vi "Kinesis - KPZ101 KSG101 - Set Position.vi"() -> ()   [LabVIEW 2012]
uses:
  U:/Kinesis LabVIEW Website Examples/Thorlabs.MotionControl.Controls.dll
  Thorlabs.MotionControl.Controls.dll
  U:/Kinesis LabVIEW Website Examples/Thorlabs.MotionControl.KCube.PiezoCLI.dll
  Thorlabs.MotionControl.KCube.PiezoCLI.dll
  U:/Kinesis LabVIEW Website Examples/Thorlabs.MotionControl.GenericPiezoCLI.dll
  Thorlabs.MotionControl.GenericPiezoCLI.dll
  U:/Kinesis LabVIEW Website Examples/ThorLabs.MotionControl.KCube.StrainGaugeCLI.dll
  ThorLabs.MotionControl.KCube.StrainGaugeCLI.dll
panel:
  in  "HubMode":i32(ring)=1 items=["AnalogueCh1"=1, "AnalogueCh2"=2, "ExtSignalSMA"=3]
  in  "stop":bool
  in  "Open Loop\nVoltage":dbl
  in  "Close Loop\n% Travel":dbl
  in  "?":bool
  in  "Zero":bool
  in  "Select Mode":bool
  in  "mode":i32(ring)=1 items=["OpenLoop"=1, "CloseLoop"=2, "OpenLoopSmooth"=3, "CloseLoopSmooth"=4]
  in  "KSG101 SerialNumber":string
  in  "KCubeStrainGaugeControl":refnum<k24>(container)
  in  "KPZ101 SerialNumber":string
  in  "KCubePiezoControl":refnum<k24>(container)
  # "Thorlabs Hardware: \nKPZ101 - K-Cube Piezo Controller\nhttps://www.thorlabs.com/newgrouppage9.cfm?objectgroup_id=2421\n\nKSG101 - K-Cube Strain Gauge Controller\nhttps://www.thorlabs.com/newgrouppage9.cfm?objectgroup_ID=242\n\nDescription: This VI will connect to & manage Closed Loop operation of the KPZ101 when used with the KSG101 Strain Gauge Controller.\nIn Closed Loop operation, as piezo actuators show a certain amount of nonlinearity, hysteresis, temperature dependence and aging, a position sensor, in this case a Strain Gauge, is read by KSG101 & feedback position information through a PI loop is managed by KPZ101 to account for this behaviour.  \nWhen in Open Loop mode, the user can adjust the Voltage of the piezo stack. \nWhen in Closed Loop mode, position can be set by use of the SetPercentageTravel() function.\n\nTo explore how to configure the KPZ101 for Closed Loop operation, plaese visit the KPZ101 User Manual. \n https://www.thorlabs.com/thorproduct.cfm?partnumber=KPZ101\n\nInstructions:\n1) Connect your KPZ101 & KSG101 devices to your PC & power each device ensuring these are correctly interconnected. Depending on whether these are connected through the KCH*** K-Cube Hub or via SMA cable will impact the choice of settings below. \nFor full device setup, the device product manual can be found on our website here. - https://www.thorlabs.com/thorproduct.cfm?partnumber=KPZ101\n2) Enter the device serial numbers below.\n3) Click 'Run' in the LabVIEW Toolbar.\n4) Ensure the HubMode is set correctly depending on how your KPZ101 & KSG101 are connected.\n5) Zero each device using the ZERO button.\n6) To end the program, click END PROGRAM."
  # "Notes:"
  # "- Ensure that the appropriate .DLLs are copied into your Project Folder. Check that the correct bit type are used depending on your version of LabVIEW\ni.e. 32-bit or 64-bit.\n\n\n\n\n\n\n\n\n\n\n\n\n\n\n- Open the example VI through the LabVIEW Project Explorer to correctly load the User Interface from Thorlabs.MotionControl.Controls.dll."
  # "Example Image of .NET Controller - VI opened via Project Explorer/ not opened via Project Explorer"
  # "VI Not Opened via Project Explorer"
  # "VI Opened via Project Explorer"
  # "- To explore the range of methods available, please visit the .NET API, included with your Kinesis software.\n\n- For tips on building your own VIs with Thorlabs Motion Control Hardware, please see our LabVIEW Guide here.\nhttps://www.thorlabs.com/newgrouppage9.cfm?objectgroup_id=10285"
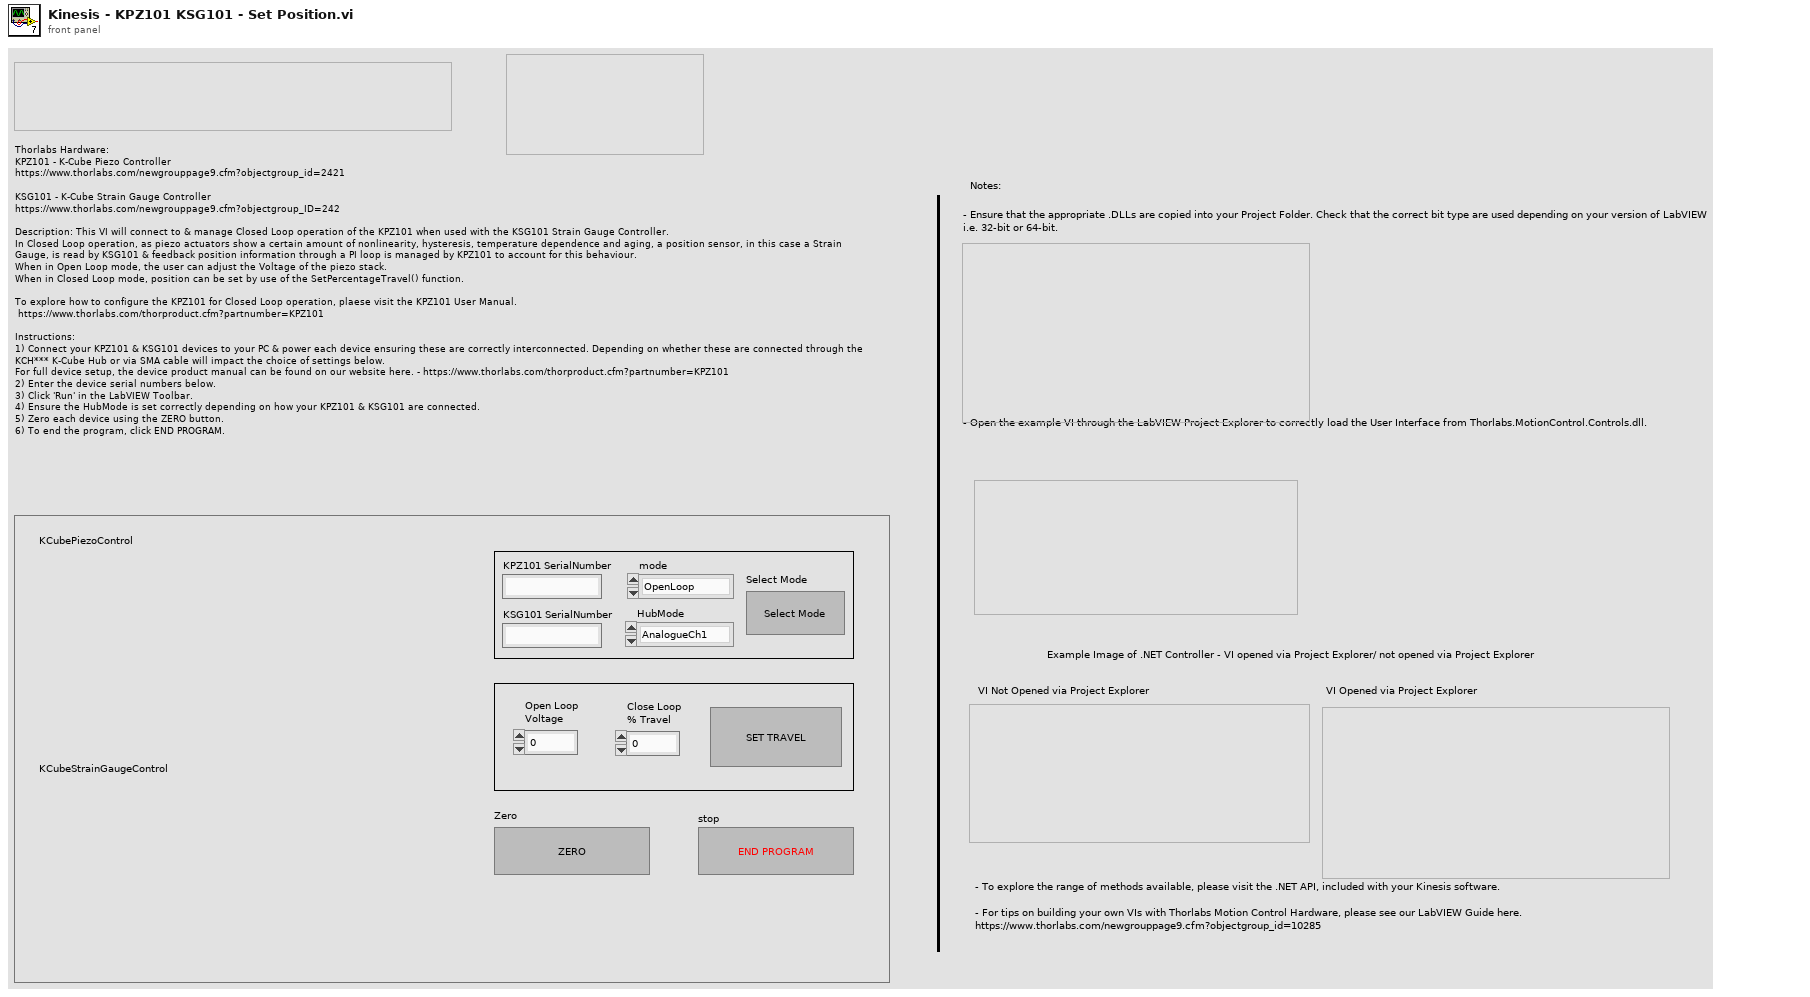
[diagram p1: front panel]
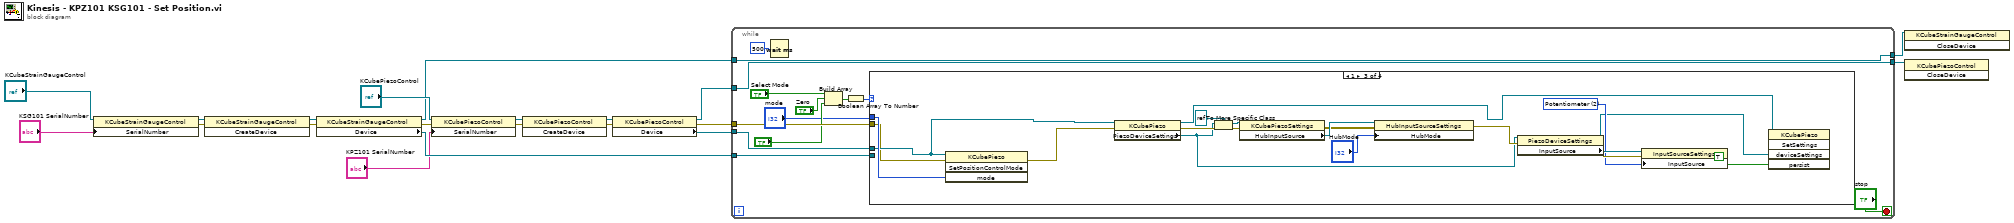
[diagram p0: block diagram]
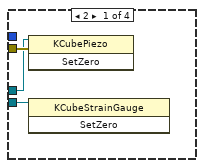
[diagram p2: hidden frame]
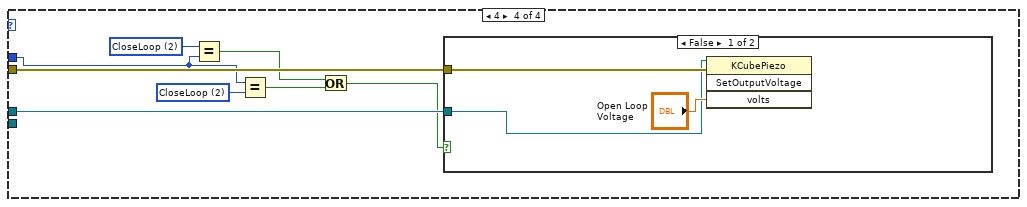
[diagram p4: hidden frame]
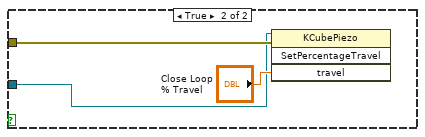
[diagram p5: hidden frame]
diagram:
  n1 = property class="KCubeStrainGaugeControl"(reference="KCubeStrainGaugeControl", "SerialNumber"="KSG101 SerialNumber") -> (reference out=w14:refnum<k24>, error out=w13:errorcluster)  [unwired: 1 in]
  n2 = invoke class="KCubeStrainGaugeControl" method="CreateDevice"(reference=w14, error in=w13) -> (reference out=w12:refnum<k24>, error out=w11:errorcluster)  [unwired: 1 in, 1 out]
  n3 = property class="KCubeStrainGaugeControl"(reference=w12, error in=w11) -> (reference out=w1:refnum<k24>, error out=w9:errorcluster, "Device"=w10:refnum<k24>)
  n4 = property class="KCubePiezoControl"(reference="KCubePiezoControl", error in=w9, "SerialNumber"="KPZ101 SerialNumber") -> (reference out=w17:refnum<k24>, error out=w8:errorcluster)
  n5 = invoke class="KCubePiezoControl" method="CreateDevice"(reference=w17, error in=w8) -> (reference out=w20:refnum<k24>, error out=w19:errorcluster)  [unwired: 1 in, 1 out]
  n6 = property class="KCubePiezoControl"(reference=w20, error in=w19) -> (reference out=w3:refnum<k24>, error out=w7:errorcluster, "Device"=w5:refnum<k24>)
  n7 = while {
    tunnel: w10 -> [w33]
    tunnel: w7 -> [w30]
    tunnel: w5 -> [w24]
    tunnel: [w23] -> w4
    tunnel: w3 -> [w23]
    tunnel: [w22] -> w2
    tunnel: w1 -> [w22]
    stop <- "stop" stop-if-true
    n8 = Wait (ms)(milliseconds to wait=u32 500) -> ()  [unwired: 1 out]
    n9 = Build Array("Select Mode", "Zero", "?") -> (w28:bool[])
    n10 = Boolean Array To Number(Boolean array=w28) -> (number=w26:u32)
    n11 = case shown="1" w26 {
      tunnel: w33 -> [w36 _ _ _]
      tunnel: "mode" -> [_ _ w42 w60]
      tunnel: w30 -> [w35 _ w38 w63]
      tunnel: w24 -> [w34 _ w39 w62]
      frame 2 {
        n12 = invoke class="KCubePiezo" method="SetZero"(reference=w34, error in=w35) -> ()  [unwired: 1 in, 3 out]
        n13 = invoke class="KCubeStrainGauge" method="SetZero"(reference=w36) -> ()  [unwired: 2 in, 3 out]
      }
      frame 0, Default {
      }
      frame 1 {
        w46 = 2 items=["SoftwareOnly", "ExternalSignal", "Potentiometer"] ("InputSource")
        n14 = invoke class="KCubePiezo" method="SetPositionControlMode"(reference=w39, error in=w38, "mode"=w42) -> (error out=w37:errorcluster)  [unwired: 1 in, 3 out]
        n15 = property class="KCubePiezo"(reference=w39, error in=w37) -> (reference out=w43:refnum<k24>, error out=w50:errorcluster, "PiezoDeviceSettings"=w41:refnum<k24>)
        n16 = To More Specific Class(target class=refnum<k24> refnum, reference=w41, error in=w50) -> (specific class reference=w53:refnum<k24>, error out=w49:errorcluster)
        n17 = property class="KCubePiezoSettings"(reference=w53, error in=w49) -> (error out=w48:errorcluster, "HubInputSource"=w51:refnum<k24>)  [unwired: 1 out]
        n18 = property class="HubInputSourceSettings"(reference=w51, error in=w48, "HubMode"="HubMode") -> (error out=w44:errorcluster)  [unwired: 1 out]
        n19 = property class="PiezoDeviceSettings"(reference=w41, error in=w44) -> (reference out=w40:refnum<k24>, error out=w54:errorcluster, "InputSource"=w55:refnum<k24>)
        n20 = property class="InputSourceSettings"(reference=w55, error in=w54, "InputSource"=w46) -> ()  [unwired: 2 out]
        n21 = invoke class="KCubePiezo" method="SetSettings"(reference=w43, "deviceSettings"=w40, "persist"=TRUE) -> ()  [unwired: 2 in, 5 out]
      }
      frame 4 {
        w59 = 2 items=["OpenLoop"=1, "CloseLoop"=2, "OpenLoopSmooth"=3, "CloseLoopSmooth"=4] ("mode")
        w61 = 2 items=["OpenLoop"=1, "CloseLoop"=2, "OpenLoopSmooth"=3, "CloseLoopSmooth"=4] ("mode")
        n22 = Equal?(x=w61, y=w60) -> (x = y?=w58:bool)
        n23 = Equal?(x=w60, y=w59) -> (x = y?=w57:bool)
        n24 = Or(x=w58, y=w57) -> (x .or. y?=w56:bool)
        n25 = case shown="False" w56 {
          tunnel: w63 -> [w65 w68]
          tunnel: w62 -> [w64 w67]
          frame False {
            n26 = invoke class="KCubePiezo" method="SetOutputVoltage"(reference=w64, error in=w65, "volts"="Open Loop\nVoltage") -> ()  [unwired: 1 in, 4 out]
          }
          frame True {
            n27 = invoke class="KCubePiezo" method="SetPercentageTravel"(reference=w67, error in=w68, "travel"="Close Loop\n% Travel") -> ()  [unwired: 1 in, 4 out]
          }
        }
      }
    }
  }
  n28 = invoke class="KCubeStrainGaugeControl" method="CloseDevice"(reference=w2) -> ()  [unwired: 2 in, 3 out]
  n29 = invoke class="KCubePiezoControl" method="CloseDevice"(reference=w4) -> ()  [unwired: 2 in, 3 out]
